vi "Reset.vi"(8 "error in (no error)":errorcluster, 10 "Message in":refnum<class "ResetMessage.lvclass">, 11 "Murmex in":refnum<class "ServiceManager.lvclass">) -> (0 "error out":errorcluster, 3 "Murmex out":refnum<class "ServiceManager.lvclass">)   [LabVIEW 2012, in "ServiceManager.lvclass"]
doc: "The reset method processes the command 'reset'. \n\nResets the internal state of the component (without performing a full initialisation). This could be resetting hardware, or private data to default values."
uses:
  ServiceManager.lvclass
  Murmex/LabVIEW/Murmex/ResetMessage/ResetMessage.lvclass
  Murmex/LabVIEW/Murmex/Murmex/Murmex.lvclass
  Murmex/LabVIEW/Murmex/InitialiseMessage/InitialiseMessage.lvclass
panel:
  # "This method is called when the RESET\ntrigger is sent. \n\nOverride this method when your component needs to\nrespond to this trigger. \n\nCall parent for proper implementation"
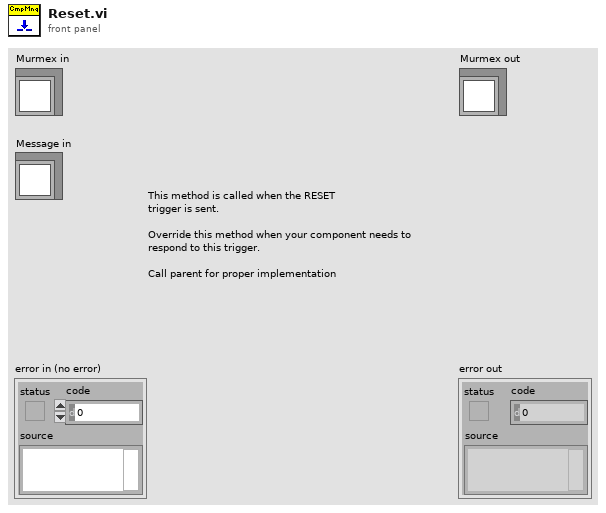
[diagram p1: front panel]
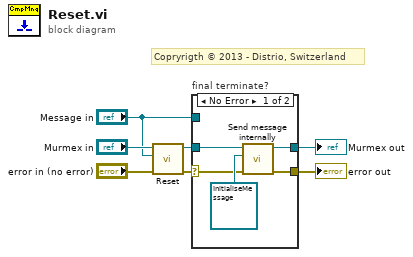
[diagram p0: block diagram]
diagram:
  # "Copryrigth © 2013 - Distrio, Switzerland"
  n1 = call-parent "Reset.vi"("error in (no error)"="error in (no error)", "Message in"="Message in", "Murmex in"="Murmex in") -> ("error out"=w4:errorcluster, "Murmex out"=w5:refnum<class "ServiceManager.lvclass">)  [unwired: 7 in]
  n2 = case "final terminate?" shown="No Error" w4 {
    selector: w4 -> [w8 w13]
    tunnel: w5 -> [w12 w14]
    tunnel: [w10 w14] -> w2
    tunnel: [w11 w13] -> w3
    tunnel: "Message in" -> [_ _]
    frame No Error {
      n3 = call "Send message internally.vi"("error in (no error)"=w8, "Message"=refnum<class "InitialiseMessage.lvclass"> refnum ("InitialiseMessage.lvclass"), "Murmex in"=w12) -> ("error out"=w11:errorcluster, "Murmex out"=w10:refnum<class "ServiceManager.lvclass">)  [unwired: 7 in]
    }
    frame Error {
    }
  }
  "error out" <- w3
  "Murmex out" <- w2
